vi "Doc_Builder_Create_Output_Name.vi"(10 "Section Name":string, 11 "Path":path) -> (3 "Full Report Name":path)   [LabVIEW 2019]
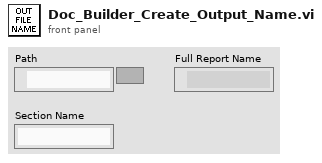
[diagram p1: front panel]
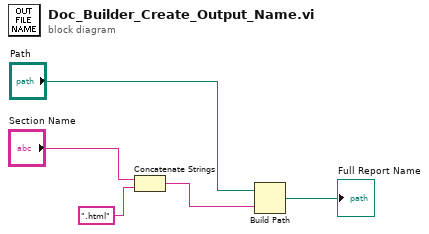
[diagram p0: block diagram]
diagram:
  n1 = Concatenate Strings("Section Name", ".html" ("string")) -> (w2:string)
  n2 = Build Path(base path="Path", name or relative path=w2) -> (appended path=→"Full Report Name":path)
